vi "MK4DueReturnState.vi"(6 "error IN":errorcluster, 8 "String IN":string) -> (0 "error out":errorcluster, 1 "Return State 2":T3=enum."Echo", 2 "OUTCONFIG":T2, 3 "outPOS":T1)   [LabVIEW 2017]
uses:
  libraryGcode/control/UartTypeDataGet.ctl
  controls/state_board_control.ctl
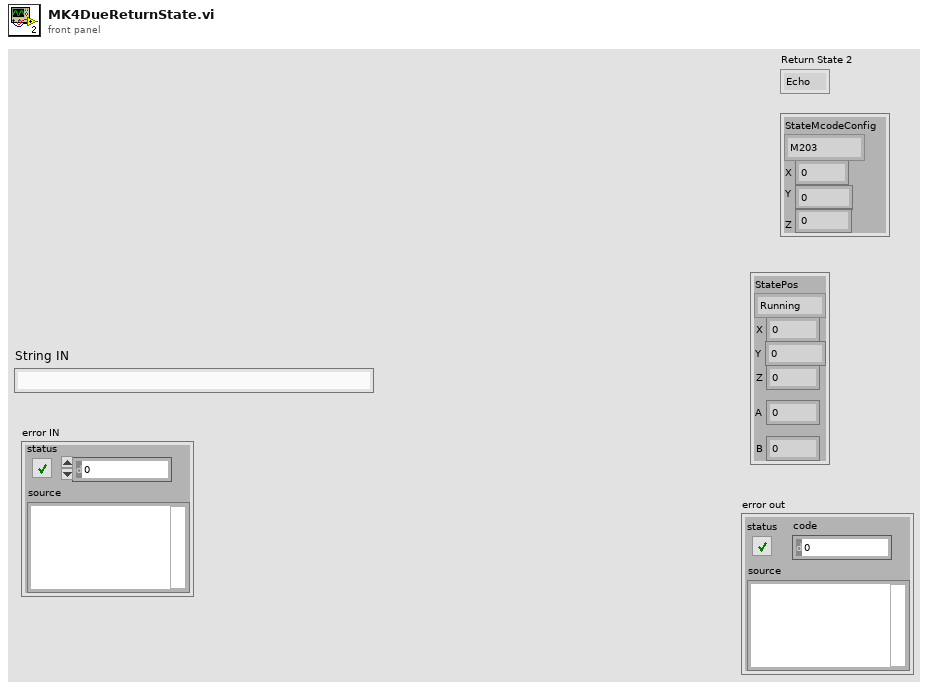
[diagram p1: front panel]
types:
  T1 = cluster{"StatePos":enum16{"Running", "Waiting", "Pos", "IDLE"}, "X":dbl, "Z":dbl, "Y":dbl, "A":dbl, "B":dbl}
  T2 = cluster{"StateMcodeConfig":enum16{"M203", "M201", "M92", "M3001", "M204"}, "X":dbl, "Y":dbl, "Z":dbl}
  T3 = typedef "UartTypeDataGet.ctl" = enum16{"Pos", "Config", "Echo", "OK", "Step", "Error"}
  T4 = typedef "state_board_control.ctl" = enum16{"Running", "Waiting", "Pos", "IDLE"}
  T5 = cluster{"StateMcodeConfig":enum16{"M203", "M201", "M92", "M3001", "M204"}, dbl, dbl, dbl}
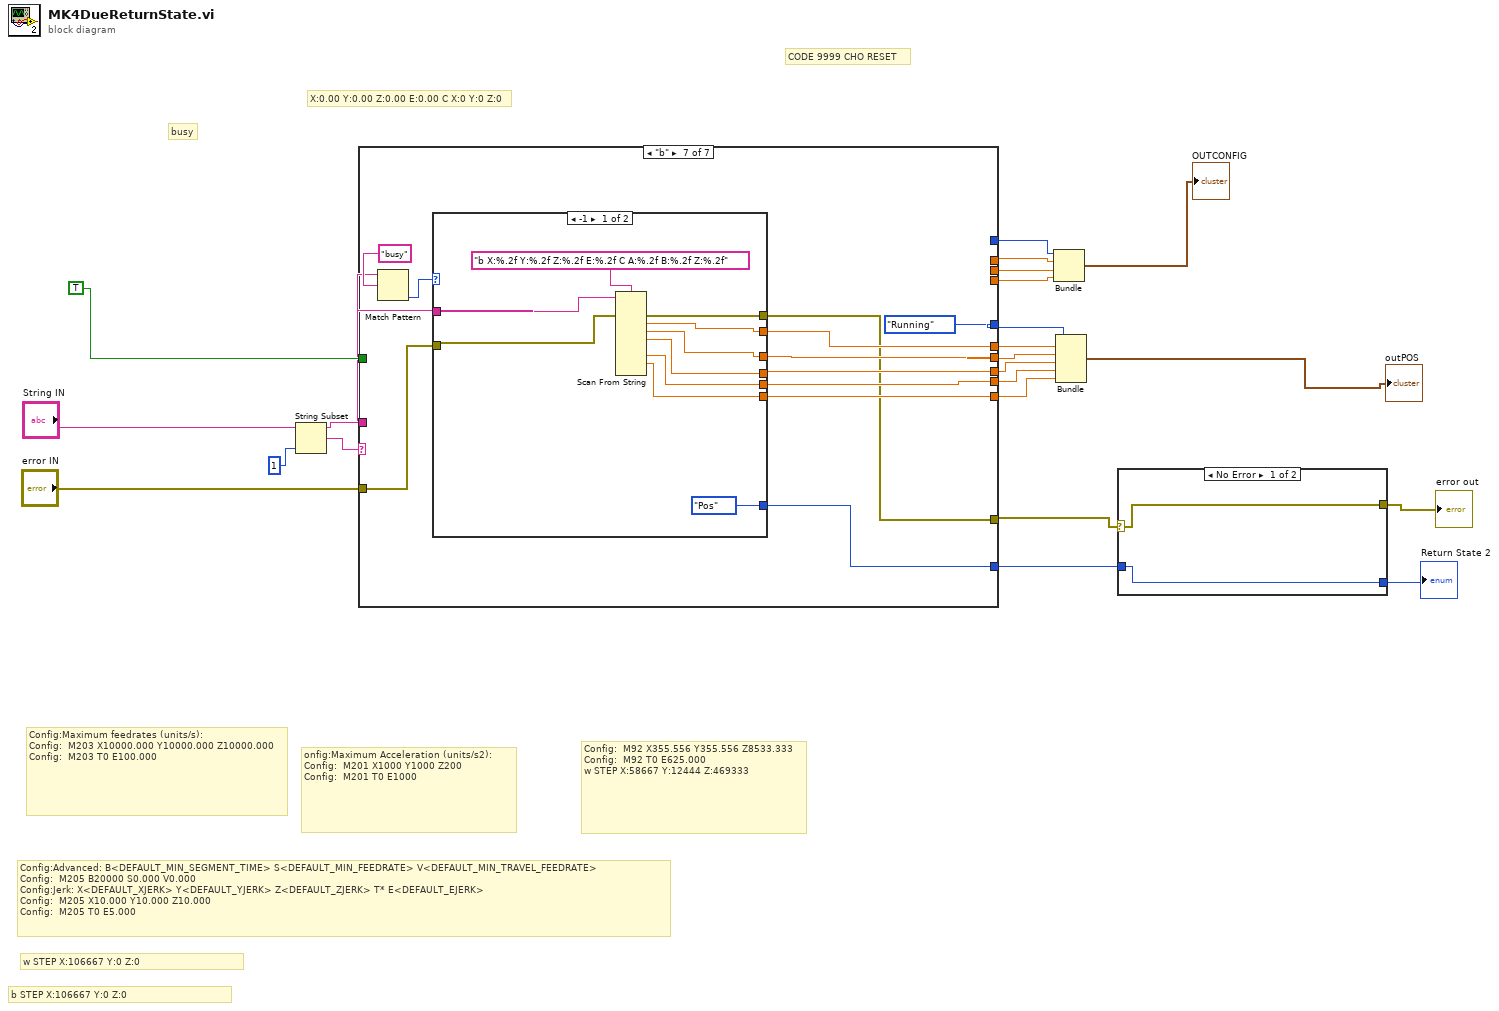
[diagram p0: block diagram]
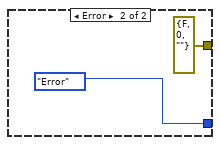
[diagram p2: hidden frame]
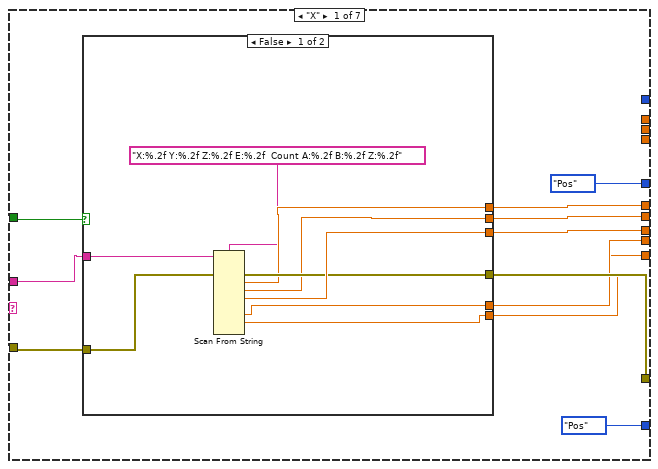
[diagram p3: hidden frame]
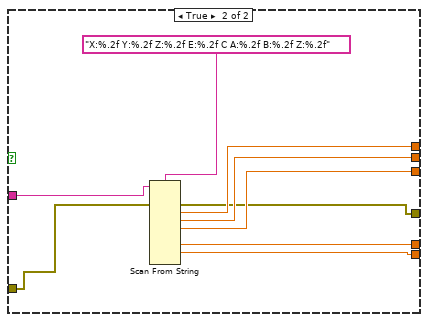
[diagram p4: hidden frame]
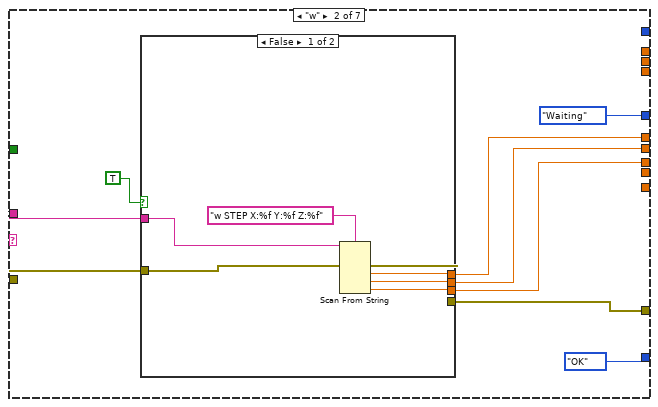
[diagram p5: hidden frame]
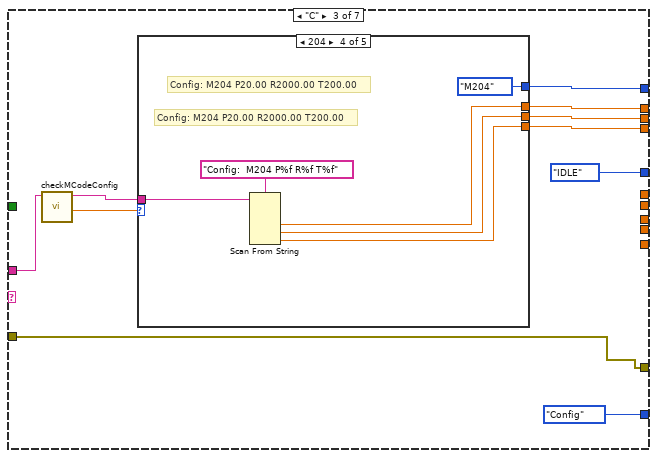
[diagram p7: hidden frame]
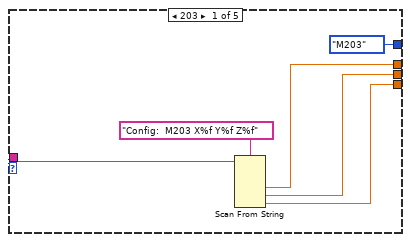
[diagram p8: hidden frame]
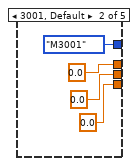
[diagram p9: hidden frame]
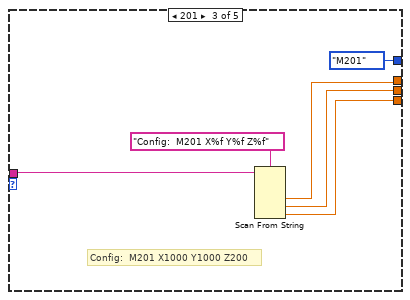
[diagram p10: hidden frame]
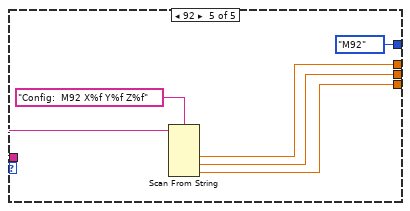
[diagram p11: hidden frame]
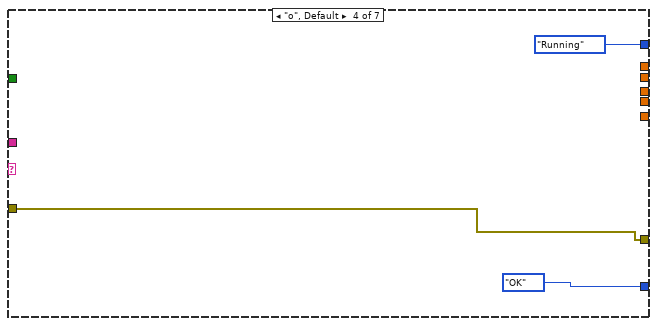
[diagram p12: hidden frame]
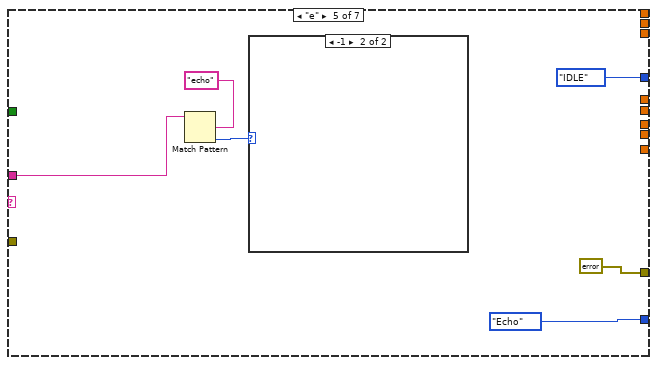
[diagram p13: hidden frame]
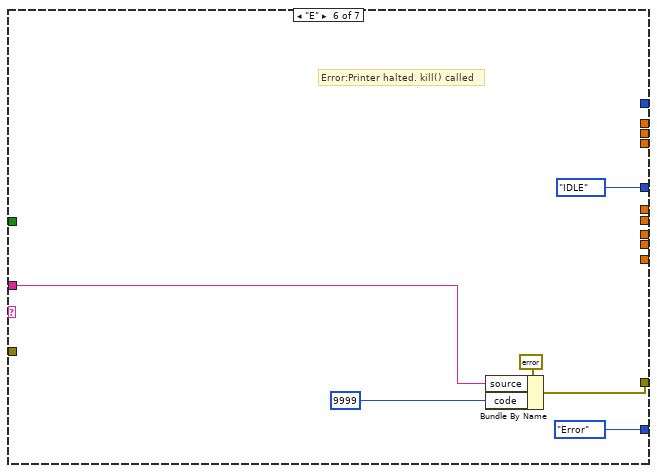
[diagram p15: hidden frame]
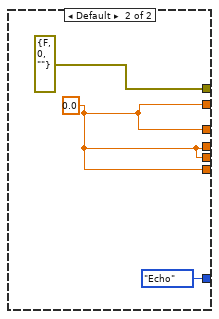
[diagram p16: hidden frame]
diagram:
  # "CODE 9999 CHO RESET"
  # "X:0.00 Y:0.00 Z:0.00 E:0.00 C X:0 Y:0 Z:0"
  # "busy"
  # "b STEP X:106667 Y:0 Z:0"
  # "Config:Advanced: B<DEFAULT_MIN_SEGMENT_TIME> S<DEFAULT_MIN_FEEDRATE> V<DEFAULT_MIN_TRAVEL_FEEDRATE>\nConfig:  M205 B20000 S0.000 V0.000\nConfig:Jerk: X<DEFAULT_XJERK> Y<DEFAULT_YJERK> Z<DEFAULT_ZJERK> T* E<DEFAULT_EJERK>\nConfig:  M205 X10.000 Y10.000 Z10.000\nConfig:  M205 T0 E5.000"
  # "Config:  M92 X355.556 Y355.556 Z8533.333\nConfig:  M92 T0 E625.000\nw STEP X:58667 Y:12444 Z:469333"
  # "onfig:Maximum Acceleration (units/s2):\nConfig:  M201 X1000 Y1000 Z200\nConfig:  M201 T0 E1000"
  # "Config:Maximum feedrates (units/s):\nConfig:  M203 X10000.000 Y10000.000 Z10000.000\nConfig:  M203 T0 E100.000"
  # "w STEP X:106667 Y:0 Z:0"
  n1 = String Subset(string="String IN", length (rest)=1 ("length (rest)")) -> (substring=w7:string)  [unwired: 1 in]
  n2 = case shown="\"b\"" w7 {
    tunnel: [state_board_control."Pos" ("Enum") state_board_control."Waiting" ("Enum") state_board_control."IDLE" ("Enum") state_board_control."Running" ("Enum") enum16{"Running", "Waiting", "Pos", "IDLE"}."IDLE" ("Enum") state_board_control."IDLE" ("Enum") state_board_control."Running" ("Enum")] -> w20
    tunnel: [w28 w58 _ _ _ _ w128] -> w17
    tunnel: [w27 w57 _ _ _ _ w129] -> w16
    tunnel: [w32 w56 _ _ _ _ w130] -> w1
    tunnel: "error IN" -> [w31 w59 w68 w106 _ _ w127]
    tunnel: [w30 w55 w68 w106 errorcluster {"status"=FALSE, "code"=0, "source"=""} ("error IO") w118 w121] -> w11
    tunnel: [_ _ w76 _ _ _ _] -> w13
    tunnel: [_ _ w75 _ _ _ _] -> w14
    tunnel: [_ _ w74 _ _ _ _] -> w15
    tunnel: [_ _ w73 _ _ _ _] -> w12
    tunnel: [UartTypeDataGet."Pos" ("Return State") UartTypeDataGet."OK" ("Return State") UartTypeDataGet."Config" ("Return State") UartTypeDataGet."OK" ("Return State") UartTypeDataGet."Echo" ("Return State") UartTypeDataGet."Error" ("Return State") w126] -> w9
    tunnel: "String IN" -> [w22 w53 w70 _ w109 w115 w125]
    tunnel: TRUE -> [w25 _ _ _ _ _ _]
    tunnel: [w24 _ _ _ _ _ w123] -> w5
    tunnel: [w23 _ _ _ _ _ w122] -> w4
    frame "X" {
      n3 = case shown="False" w25 {
        tunnel: [w41 w46] -> w32
        tunnel: w31 -> [w40 w45]
        tunnel: [w39 w44] -> w30
        tunnel: [w38 w48] -> w28
        tunnel: [w37 w47] -> w27
        tunnel: w22 -> [w36 w49]
        tunnel: [w33 w43] -> w24
        tunnel: [w34 w42] -> w23
        frame False {
          n4 = Scan From String(format string="X:%.2f Y:%.2f Z:%.2f E:%.2f  Count A:%.2f B:%.2f Z:%.2f", input string=w36, error in=w40) -> (error out=w39:errorcluster, output 1=w38:dbl, output 2=w37:dbl, output 3=w41:dbl, output 5=w33:dbl, output 6=w34:dbl)  [unwired: 10 in, 2 out]
        }
        frame True {
          n5 = Scan From String(format string="X:%.2f Y:%.2f Z:%.2f E:%.2f C A:%.2f B:%.2f Z:%.2f", input string=w49, error in=w45) -> (error out=w44:errorcluster, output 1=w48:dbl, output 2=w47:dbl, output 3=w46:dbl, output 5=w43:dbl, output 6=w42:dbl)  [unwired: 10 in, 2 out]
        }
      }
    }
    frame "w" {
      n6 = case shown="False" TRUE {
        tunnel: w59 -> [w65 w67]
        tunnel: [w64 _] -> w58
        tunnel: [w63 _] -> w57
        tunnel: [w62 _] -> w56
        tunnel: [w61 w67] -> w55
        tunnel: w53 -> [w60 _]
        frame False {
          n7 = Scan From String(format string="w STEP X:%f Y:%f Z:%f", input string=w60, error in=w65) -> (error out=w61:errorcluster, output 1=w64:dbl, output 2=w63:dbl, output 3=w62:dbl)  [unwired: 4 in, 2 out]
        }
        frame True {
        }
      }
    }
    frame "C" {
      n8 = call "checkMCodeConfig.vi"("INPUT"=w70) -> ("MCODE"=w69:dbl, "OUTPUT"=w77:string)  [unwired: 9 in]
      n9 = case shown="204" w69 {
        tunnel: w77 -> [w82 _ w92 w98 w104]
        tunnel: [w81 0.0 w91 w96 w103] -> w76
        tunnel: [w80 0.0 w88 w95 w102] -> w75
        tunnel: [w79 0.0 w90 w94 w101] -> w74
        tunnel: [enum16{"M203", "M201", "M92", "M3001", "M204"}."M203" ("StateMcodeConfig") enum16{"M203", "M201", "M92", "M3001", "M204"}."M3001" ("StateMcodeConfig") enum16{"M203", "M201", "M92", "M3001", "M204"}."M201" ("StateMcodeConfig") enum16{"M203", "M201", "M92", "M3001", "M204"}."M204" ("StateMcodeConfig") enum16{"M203", "M201", "M92", "M3001", "M204"}."M92" ("StateMcodeConfig")] -> w73
        frame 203 {
          n10 = Scan From String(format string="Config:  M203 X%f Y%f Z%f", input string=w82) -> (output 1=w81:dbl, output 2=w80:dbl, output 3=w79:dbl)  [unwired: 5 in, 3 out]
        }
        frame 3001, Default {
        }
        frame 201 {
          # "Config:  M201 X1000 Y1000 Z200"
          n11 = Scan From String(format string="Config:  M201 X%f Y%f Z%f", input string=w92) -> (output 1=w91:dbl, output 2=w88:dbl, output 3=w90:dbl)  [unwired: 5 in, 3 out]
        }
        frame 204 {
          # "Config: M204 P20.00 R2000.00 T200.00"
          # "Config: M204 P20.00 R2000.00 T200.00"
          n12 = Scan From String(format string="Config:  M204 P%f R%f T%f", input string=w98) -> (output 1=w96:dbl, output 2=w95:dbl, output 3=w94:dbl)  [unwired: 5 in, 3 out]
        }
        frame 92 {
          n13 = Scan From String(format string="Config:  M92 X%f Y%f Z%f", input string=w104) -> (output 1=w103:dbl, output 2=w102:dbl, output 3=w101:dbl)  [unwired: 5 in, 3 out]
        }
      }
    }
    frame "o", Default {
    }
    frame "e" {
      n14 = Match Pattern(string=w109, regular expression="echo") -> (offset past match=w113:i32)  [unwired: 1 in, 3 out]
      n15 = case shown="-1" w113 {
        frame Default {
        }
        frame -1 {
        }
      }
    }
    frame "E" {
      # "Error:Printer halted. kill() called"
      n16 = Bundle By Name(cluster=errorcluster {"status"=FALSE, "code"=0, "source"="REBOOT"} ("error IO"), "source"=w115, "code"=9999) -> (w118:errorcluster)
    }
    frame "b" {
      n17 = Match Pattern(string=w125, regular expression="busy") -> (offset past match=w131:i32)  [unwired: 1 in, 3 out]
      n18 = case shown="-1" w131 {
        tunnel: w127 -> [w142 _]
        tunnel: [w141 errorcluster {"status"=FALSE, "code"=0, "source"=""} ("error IO")] -> w121
        tunnel: [w137 w143] -> w129
        tunnel: [w136 w143] -> w128
        tunnel: [w138 w143] -> w130
        tunnel: w125 -> [w140 _]
        tunnel: [UartTypeDataGet."Pos" ("Return State") UartTypeDataGet."Echo" ("Return State")] -> w126
        tunnel: [w133 w143] -> w123
        tunnel: [w134 w143] -> w122
        frame -1 {
          n19 = Scan From String(format string="b X:%.2f Y:%.2f Z:%.2f E:%.2f C A:%.2f B:%.2f Z:%.2f", input string=w140, error in=w142) -> (error out=w141:errorcluster, output 1=w136:dbl, output 2=w137:dbl, output 3=w138:dbl, output 5=w133:dbl, output 6=w134:dbl)  [unwired: 10 in, 2 out]
        }
        frame Default {
          w143 = 0.0
        }
      }
    }
  }
  n20 = Bundle("StateMcodeConfig"=w12, w13, w14, w15) -> (→"OUTCONFIG":T5)  [unwired: 1 in]
  n21 = Bundle("Enum"=w20, w17, w16, w1, w5, w4) -> (→"outPOS":cluster{"Enum":T4, dbl, dbl, dbl, dbl, dbl})  [unwired: 1 in]
  n22 = case shown="No Error" w11 {
    selector: w11 -> [w147 _]
    tunnel: [w147 errorcluster {"status"=FALSE, "code"=0, "source"=""} ("error IO")] -> w19
    tunnel: w9 -> [w146 _]
    tunnel: [w146 UartTypeDataGet."Error" ("Return State")] -> w10
    frame No Error {
    }
    frame Error {
    }
  }
  "error out" <- w19
  "Return State 2" <- w10
